vi "JournalExists.vi"(4 "Visible (T)":bool=TRUE, 5 "closing behavior (leave open)":T1(ring), 7 "JournalPath":path, 8 "Error In":errorcluster, 11 "Reference In":T2) -> (0 "Error Out":errorcluster, 3 "Reference Out":T2)   [LabVIEW 2013, in "Medimatic.lvlib"]
uses:
  Medimatic.lvlib
  <userlib>/_OpenG.lib/file/file.llb/File Exists - Scalar__ogtk.vi
  <userlib>/Excel/excel.llb/excel Object Reference.ctl
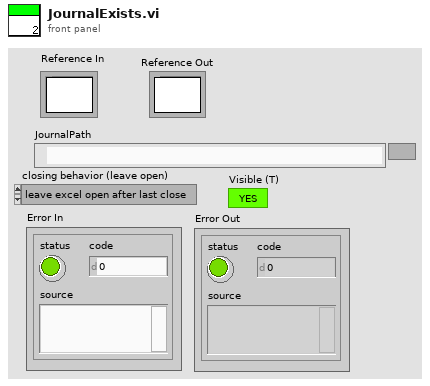
[diagram p1: front panel]
types:
  T1 = enum16{"leave excel open after last close", "close only if opened by LabVIEW", "close excel after last close"}
  T2 = typedef "excel Object Reference.ctl" = refnum<k1>
  T3 = enum16{"open workbook as template", "open workbook from file", "create new workbook"}
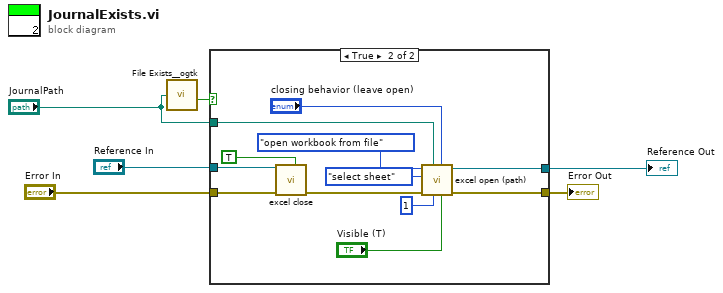
[diagram p0: block diagram]
diagram:
  n1 = call-poly <userlib>:"File Exists__ogtk.vi"("file path"="JournalPath") -> ("exists"=w6:bool)  [unwired: 6 in, 1 out]
  n2 = case shown="True" w6 {
    tunnel: "JournalPath" -> [_ w19]
    tunnel: "Error In" -> [w8 w15]
    tunnel: [w8 w14] -> w3
    tunnel: "Reference In" -> [w7 w13]
    tunnel: [w7 w12] -> w1
    frame False {
    }
    frame True {
      n3 = call <userlib>:"excel close.vi"("Close"=TRUE, "error in (no error)"=w15, "reference"=w13) -> ("error out"=w20:errorcluster)  [unwired: 8 in]
      n4 = call <userlib>:"excel open (path).vi"("Visible (T)"="Visible (T)", "closing behavior (leave open)"="closing behavior (leave open)", "worksheet_number"=u8 1, "workbook path"=w19, "error in (no error)"=w20, "select/new"=enum16{"new sheet", "select sheet"}."select sheet", "create/open template/open file"=T3."open workbook from file") -> ("error out"=w14:errorcluster, "reference"=w12:T2)  [unwired: 3 in]
    }
  }
  "Error Out" <- w3
  "Reference Out" <- w1
